vi "Field vs  IV_old_20180522.vi"() -> ()   [LabVIEW 2017]
uses:
  <vilib>/LabVIEW Targets/FPGA/cRIO/shared/nicrio_ModuleControls/nicrio_cRIO-9775_RecordDataRates4ChansRing.ctl
  <vilib>/Utility/file.llb/Write Delimited Spreadsheet (DBL).vi
  global.vi
  <resource>/objmgr/ni.dex.rc
panel:
  out "Array":dbl[](array[numeric])
  in  "Tab Control":enum32{"Field", "cRIO"}(tab)
  in  "Ramp type":string(combo)="Around origin"
  in  "Ramp up first T":bool=TRUE
  in  "Field Origin V":dbl format="%#_13g"
  in  "Field step V":dbl=0.005 format="%#_13g"
  in  "Field Radius V":dbl=1.0 format="%#_13g"
  in  "Init Ramp Time s":dbl=10.0
  in  "FIeld Scale factor":dbl=10.0
  in  "Step Ramp Time s":dbl=1.0
  in  "KEITHLEY 2400 GPIB Address":string="22"
  in  "cRIO IP":string="//172.22.11.2"
  in  "Data buffer size":i32=1000
  in  "Record Data Rate":T1=200 items=["20.000 MS/s (NI 9775)"=1, "10.00 MS/s (NI 9775)"=2, "6.667 MS/s (NI 9775)"=3, "5.000 MS/s (NI 9775)"=4, "2.500 MS/s (NI 9775)"=8, "1.667 MS/s (NI 9775)"=12, "1.250 MS/s (NI 9775)"=16, "1.000 MS/s (NI 9775)"=20, "833.333 KS/s (NI 9775)"=24, "714.286 KS/s (NI 9775)"=28, "625.000 KS/s (NI 9775)"=32, "555.556 KS/s (NI 9775)"=36, "500.000 KS/s (NI 9775)"=40, "454.545 KS/s (NI 9775)"=44, "416.667 KS/s (NI 9775)"=48, "384.615 KS/s (NI 9775)"=52, "357.143 KS/s (NI 9775)"=56, "333.333 KS/s (NI 9775)"=60, "312.500 KS/s (NI 9775)"=64, "294.118 KS/s (NI 9775)"=68, "277.778 KS/s (NI 9775)"=72, "263.158 KS/s (NI 9775)"=76, "250.000 KS/s (NI 9775)"=80, "238.095 KS/s (NI 9775)"=84, "227.273 KS/s (NI 9775)"=88, "217.391 KS/s (NI 9775)"=92, "208.333 KS/s (NI 9775)"=96, "200.000 KS/s (NI 9775)"=100, "192.308 KS/s (NI 9775)"=104, "185.185 KS/s (NI 9775)"=108, "178.571 KS/s (NI 9775)"=112, "172.414 KS/s (NI 9775)"=116, "166.667 KS/s (NI 9775)"=120, "161.290 KS/s (NI 9775)"=124, "156.250 KS/s (NI 9775)"=128, "151.515 KS/s (NI 9775)"=132, "147.059 KS/s (NI 9775)"=136, "142.857 KS/s (NI 9775)"=140, "138.889 KS/s (NI 9775)"=144, "135.135 KS/s (NI 9775)"=148, "131.579 KS/s (NI 9775)"=152, "128.205 KS/s (NI 9775)"=156, "125.000 KS/s (NI 9775)"=160, "121.951 KS/s (NI 9775)"=164, "119.048 KS/s (NI 9775)"=168, "116.279 KS/s (NI 9775)"=172, "113.636 KS/s (NI 9775)"=176, "111.111 KS/s (NI 9775)"=180, "108.696 KS/s (NI 9775)"=184, "106.383 KS/s (NI 9775)"=188, "104.167 KS/s (NI 9775)"=192, "102.041 KS/s (NI 9775)"=196, "100.000 KS/s (NI 9775)"=200, "50.000 KS/s (NI 9775)"=400, "33.333 KS/s (NI 9775)"=600, "25.000 KS/s (NI 9775)"=800, "20.000 KS/s (NI 9775)"=1000, "16.667 KS/s (NI 9775)"=1200, "14.286 KS/s (NI 9775)"=1400, "12.500 KS/s (NI 9775)"=1600, "11.111 KS/s (NI 9775)"=1800, "10.000 KS/s (NI 9775)"=2000, "9.091 KS/s (NI 9775)"=2200, "8.333 KS/s (NI 9775)"=2400, "7.692 KS/s (NI 9775)"=2600, "7.143 KS/s (NI 9775)"=2800, "6.667 KS/s (NI 9775)"=3000, "6.250 KS/s (NI 9775)"=3200, "5.882 KS/s (NI 9775)"=3400, "5.556 KS/s (NI 9775)"=3600, "5.000 KS/s (NI 9775)"=4000, "4.762 KS/s (NI 9775)"=4200, "4.545 KS/s (NI 9775)"=4400, "4.348 KS/s (NI 9775)"=4600, "4.167 KS/s (NI 9775)"=4800, "4.000 KS/s (NI 9775)"=5000, "3.846 KS/s (NI 9775)"=5200, "3.571 KS/s (NI 9775)"=5600, "3.333 KS/s (NI 9775)"=6000, "3.125 KS/s (NI 9775)"=6400, "2.941 KS/s (NI 9775)"=6800, "2.778 KS/s (NI 9775)"=7200, "2.632 KS/s (NI 9775)"=7600, "2.500 KS/s (NI 9775)"=8000, "2.381 KS/s (NI 9775)"=8400, "2.273 KS/s (NI 9775)"=8800, "2.174 KS/s (NI 9775)"=9200, "2.083 KS/s (NI 9775)"=9600, "2.000 KS/s (NI 9775)"=10000, "1.923 KS/s (NI 9775)"=10400, "1.852 KS/s (NI 9775)"=10800, "1.786 KS/s (NI 9775)"=11200, "1.724 KS/s (NI 9775)"=11600, "1.667 KS/s (NI 9775)"=12000, "1.613 KS/s (NI 9775)"=12400, "1.563 KS/s (NI 9775)"=12800, "1.515 KS/s (NI 9775)"=13200, "1.471 KS/s (NI 9775)"=13600, "1.429 KS/s (NI 9775)"=14000, "1.389 KS/s (NI 9775)"=14400, "1.351 KS/s (NI 9775)"=14800, "1.316 KS/s (NI 9775)"=15200, "1.282 KS/s (NI 9775)"=15600, "1.250 KS/s (NI 9775)"=16000, "1.220 KS/s (NI 9775)"=16400, "1.190 KS/s (NI 9775)"=16800, "1.163 KS/s (NI 9775)"=17200, "1.136 KS/s (NI 9775)"=17600, "1.111 KS/s (NI 9775)"=18000, "1.087 KS/s (NI 9775)"=18400, "1.064 KS/s (NI 9775)"=18800, "1.042 KS/s (NI 9775)"=19200, "1.020 KS/s (NI 9775)"=19600, "1.000 KS/s (NI 9775)"=20000, "0.980 KS/s (NI 9775)"=20400, "0.962 KS/s (NI 9775)"=20800, "0.943 KS/s (NI 9775)"=21200, "0.926 KS/s (NI 9775)"=21600, "0.909 KS/s (NI 9775)"=22000, "0.893 KS/s (NI 9775)"=22400, "0.877 KS/s (NI 9775)"=22800, "0.862 KS/s (NI 9775)"=23200, "0.847 KS/s (NI 9775)"=23600, "0.833 KS/s (NI 9775)"=24000, "0.820 KS/s (NI 9775)"=24400, "0.806 KS/s (NI 9775)"=24800, "0.794 KS/s (NI 9775)"=25200, "0.781 KS/s (NI 9775)"=25600, "0.694 KS/s (NI 9775)"=28800, "0.625 KS/s (NI 9775)"=32000, "0.568 KS/s (NI 9775)"=35200, "0.521 KS/s (NI 9775)"=38400, "0.446 KS/s (NI 9775)"=44800, "0.391 KS/s (NI 9775)"=51200, "0.347 KS/s (NI 9775)"=57600, "0.313 KS/s (NI 9775)"=64000]
  in  "Gate wait time us":u32=150
  in  "Record Samples":u32=5000
  in  "Current Scale factor":dbl=5.0
  in  "Average num":i32=10
  in  "Voltage Scale factor":dbl=0.0001
  in  "Stop loop":bool
  out "Current Field mT":dbl=-0.050000000000000044
  out "Current Field V":dbl=-0.0050000000000000044
  in  "Name":string="book381"
  in  "Contour plot folder":path=path "C:/Users/gyue/Box Sync/Guang Yue/data/Contour plot"
  out "IV parameters":T2={"Records Num"=1, "AI Trigger Configuration"={"Trigger Slope"=enum."Positive", "Trigger Level"=0.10009765625, "Hystesis Value"=0.094970703125, "AI Channel"=0}, "Record PreTrigger Samples"=1, "Record Samples"=5000, "Ic Cut off or curve"=FALSE, "Gate wait time us"=150, "Record Data Rate"=200} {"Record Data Rate" items=["20.000 MS/s (NI 9775)"=1, "10.00 MS/s (NI 9775)"=2, "6.667 MS/s (NI 9775)"=3, "5.000 MS/s (NI 9775)"=4, "2.500 MS/s (NI 9775)"=8, "1.667 MS/s (NI 9775)"=12, "1.250 MS/s (NI 9775)"=16, "1.000 MS/s (NI 9775)"=20, "833.333 KS/s (NI 9775)"=24, "714.286 KS/s (NI 9775)"=28, "625.000 KS/s (NI 9775)"=32, "555.556 KS/s (NI 9775)"=36, "500.000 KS/s (NI 9775)"=40, "454.545 KS/s (NI 9775)"=44, "416.667 KS/s (NI 9775)"=48, "384.615 KS/s (NI 9775)"=52, "357.143 KS/s (NI 9775)"=56, "333.333 KS/s (NI 9775)"=60, "312.500 KS/s (NI 9775)"=64, "294.118 KS/s (NI 9775)"=68, "277.778 KS/s (NI 9775)"=72, "263.158 KS/s (NI 9775)"=76, "250.000 KS/s (NI 9775)"=80, "238.095 KS/s (NI 9775)"=84, "227.273 KS/s (NI 9775)"=88, "217.391 KS/s (NI 9775)"=92, "208.333 KS/s (NI 9775)"=96, "200.000 KS/s (NI 9775)"=100, "192.308 KS/s (NI 9775)"=104, "185.185 KS/s (NI 9775)"=108, "178.571 KS/s (NI 9775)"=112, "172.414 KS/s (NI 9775)"=116, "166.667 KS/s (NI 9775)"=120, "161.290 KS/s (NI 9775)"=124, "156.250 KS/s (NI 9775)"=128, "151.515 KS/s (NI 9775)"=132, "147.059 KS/s (NI 9775)"=136, "142.857 KS/s (NI 9775)"=140, "138.889 KS/s (NI 9775)"=144, "135.135 KS/s (NI 9775)"=148, "131.579 KS/s (NI 9775)"=152, "128.205 KS/s (NI 9775)"=156, "125.000 KS/s (NI 9775)"=160, "121.951 KS/s (NI 9775)"=164, "119.048 KS/s (NI 9775)"=168, "116.279 KS/s (NI 9775)"=172, "113.636 KS/s (NI 9775)"=176, "111.111 KS/s (NI 9775)"=180, "108.696 KS/s (NI 9775)"=184, "106.383 KS/s (NI 9775)"=188, "104.167 KS/s (NI 9775)"=192, "102.041 KS/s (NI 9775)"=196, "100.000 KS/s (NI 9775)"=200, "50.000 KS/s (NI 9775)"=400, "33.333 KS/s (NI 9775)"=600, "25.000 KS/s (NI 9775)"=800, "20.000 KS/s (NI 9775)"=1000, "16.667 KS/s (NI 9775)"=1200, "14.286 KS/s (NI 9775)"=1400, "12.500 KS/s (NI 9775)"=1600, "11.111 KS/s (NI 9775)"=1800, "10.000 KS/s (NI 9775)"=2000, "9.091 KS/s (NI 9775)"=2200, "8.333 KS/s (NI 9775)"=2400, "7.692 KS/s (NI 9775)"=2600, "7.143 KS/s (NI 9775)"=2800, "6.667 KS/s (NI 9775)"=3000, "6.250 KS/s (NI 9775)"=3200, "5.882 KS/s (NI 9775)"=3400, "5.556 KS/s (NI 9775)"=3600, "5.000 KS/s (NI 9775)"=4000, "4.762 KS/s (NI 9775)"=4200, "4.545 KS/s (NI 9775)"=4400, "4.348 KS/s (NI 9775)"=4600, "4.167 KS/s (NI 9775)"=4800, "4.000 KS/s (NI 9775)"=5000, "3.846 KS/s (NI 9775)"=5200, "3.571 KS/s (NI 9775)"=5600, "3.333 KS/s (NI 9775)"=6000, "3.125 KS/s (NI 9775)"=6400, "2.941 KS/s (NI 9775)"=6800, "2.778 KS/s (NI 9775)"=7200, "2.632 KS/s (NI 9775)"=7600, "2.500 KS/s (NI 9775)"=8000, "2.381 KS/s (NI 9775)"=8400, "2.273 KS/s (NI 9775)"=8800, "2.174 KS/s (NI 9775)"=9200, "2.083 KS/s (NI 9775)"=9600, "2.000 KS/s (NI 9775)"=10000, "1.923 KS/s (NI 9775)"=10400, "1.852 KS/s (NI 9775)"=10800, "1.786 KS/s (NI 9775)"=11200, "1.724 KS/s (NI 9775)"=11600, "1.667 KS/s (NI 9775)"=12000, "1.613 KS/s (NI 9775)"=12400, "1.563 KS/s (NI 9775)"=12800, "1.515 KS/s (NI 9775)"=13200, "1.471 KS/s (NI 9775)"=13600, "1.429 KS/s (NI 9775)"=14000, "1.389 KS/s (NI 9775)"=14400, "1.351 KS/s (NI 9775)"=14800, "1.316 KS/s (NI 9775)"=15200, "1.282 KS/s (NI 9775)"=15600, "1.250 KS/s (NI 9775)"=16000, "1.220 KS/s (NI 9775)"=16400, "1.190 KS/s (NI 9775)"=16800, "1.163 KS/s (NI 9775)"=17200, "1.136 KS/s (NI 9775)"=17600, "1.111 KS/s (NI 9775)"=18000, "1.087 KS/s (NI 9775)"=18400, "1.064 KS/s (NI 9775)"=18800, "1.042 KS/s (NI 9775)"=19200, "1.020 KS/s (NI 9775)"=19600, "1.000 KS/s (NI 9775)"=20000, "0.980 KS/s (NI 9775)"=20400, "0.962 KS/s (NI 9775)"=20800, "0.943 KS/s (NI 9775)"=21200, "0.926 KS/s (NI 9775)"=21600, "0.909 KS/s (NI 9775)"=22000, "0.893 KS/s (NI 9775)"=22400, "0.877 KS/s (NI 9775)"=22800, "0.862 KS/s (NI 9775)"=23200, "0.847 KS/s (NI 9775)"=23600, "0.833 KS/s (NI 9775)"=24000, "0.820 KS/s (NI 9775)"=24400, "0.806 KS/s (NI 9775)"=24800, "0.794 KS/s (NI 9775)"=25200, "0.781 KS/s (NI 9775)"=25600, "0.694 KS/s (NI 9775)"=28800, "0.625 KS/s (NI 9775)"=32000, "0.568 KS/s (NI 9775)"=35200, "0.521 KS/s (NI 9775)"=38400, "0.446 KS/s (NI 9775)"=44800, "0.391 KS/s (NI 9775)"=51200, "0.347 KS/s (NI 9775)"=57600, "0.313 KS/s (NI 9775)"=64000]}
  out "IV curve":cluster{"Y":dbl[], "Y":dbl[]}[](graph)
  in  "stop":bool
  out "error out":errorcluster={"status"=FALSE, "code"=180121605, "source"="Shared Variable in Field vs  IV.vi<APPEND>\nThis error or warning occurred while writing the following Shared Variable:\n\\\\NI-cRIO-9063-01bc8cc6\\network varibles\\RT Stop\n\\\\172.22.11.2\\network varibles\\RT Stop"}
  # "Voltage x factor=mT"
  # "Voltage x factor=uA"
  # "Voltage x factor=uA"
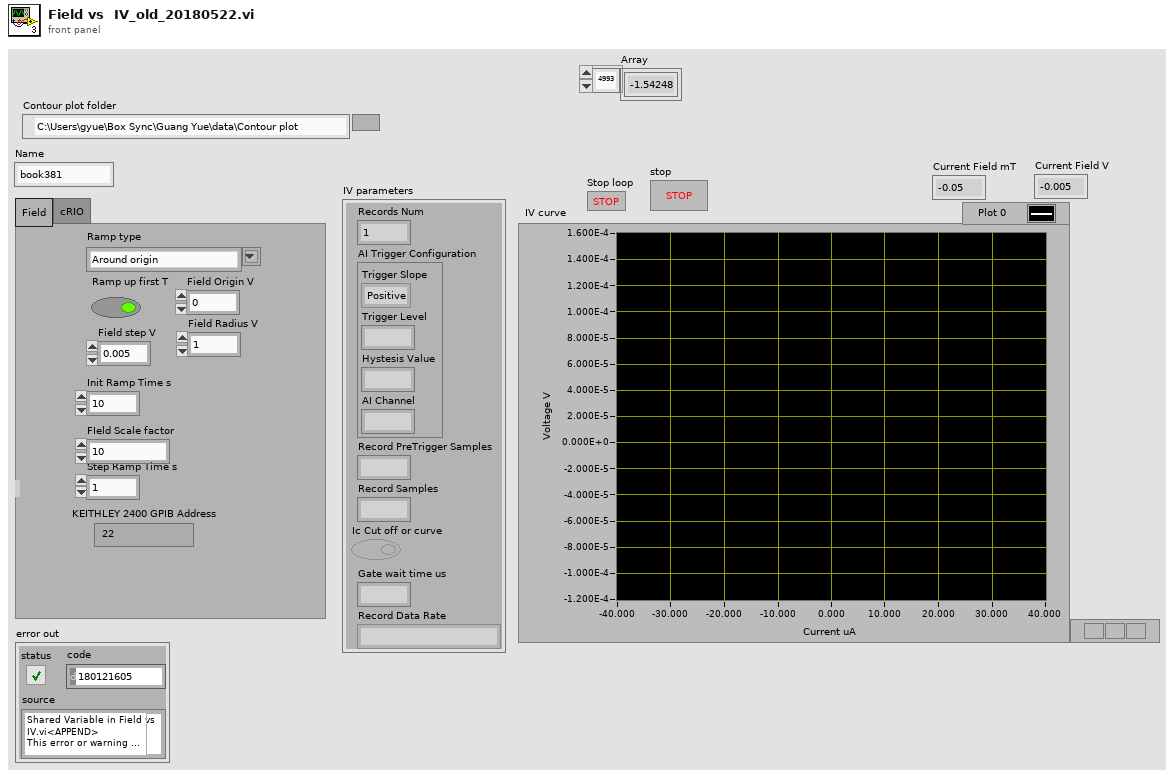
[diagram p1: front panel]
types:
  T1 = typedef "nicrio_cRIO-9775_RecordDataRates4ChansRing.ctl" = u16
  T2 = cluster{"Records Num":i32, "AI Trigger Configuration":cluster{"Trigger Slope":enum8{"Positive", "Negative"}, "Trigger Level":fxp<+/-,17,5>, "Hystesis Value":fxp<+,16,4>, "AI Channel":u8}, "Record PreTrigger Samples":u32, "Record Samples":u32, "Ic Cut off or curve":bool, "Gate wait time us":u32, "Record Data Rate":T1}
  T3 = cluster{"Trigger Slope":enum8{"Positive", "Negative"}, "Trigger Level":fxp<+/-,17,5>, "Hystesis Value":fxp<+,16,4>, "AI Channel":u8}
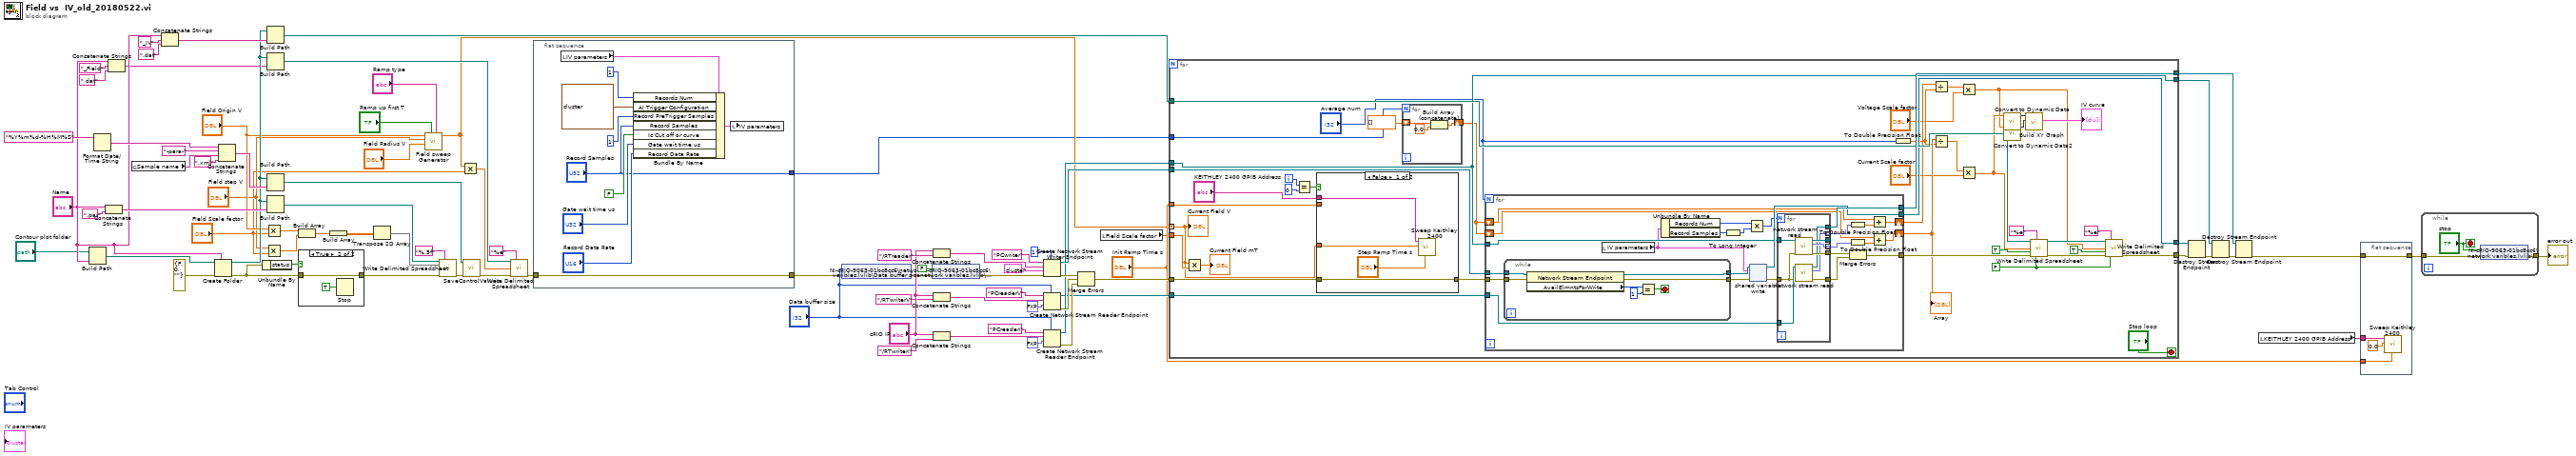
[diagram p0: block diagram]
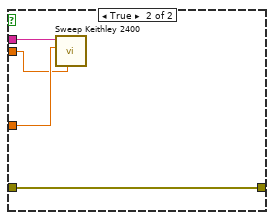
[diagram p3: hidden frame]
diagram:
  n1 = Build Path(base path="Contour plot folder", name or relative path="Name") -> (appended path=w37:path)
  n2 = Format Date/Time String(time format string (%c)="%Y%m%d-%H%M%S") -> (date/time string=w32:string)  [unwired: 2 in]
  n3 = Concatenate Strings("Name", ".par" ("string")) -> (w44:string)
  n4 = Concatenate Strings("Name", "_Field" ("string"), ".dat" ("string")) -> (w21:string)
  n5 = global read "global.vi" "Sample name"() -> (w31:string)
  n6 = Concatenate Strings("Name", "_IV" ("string"), ".dat" ("string")) -> (w38:string)
  n7 = Create Folder(prompt (Create Folder)="Name", path (use dialog)=w37, error in=errorcluster {"status"=FALSE, "code"=0, "source"=""}) -> (created path=w22:path, error out=w34:errorcluster)  [unwired: 1 out]
  n8 = Concatenate Strings(w32, "-para-" ("string"), w31, ".xml" ("string")) -> (w48:string)
  n9 = Unbundle By Name(w34) -> ("status"=w35:bool)
  n10 = Multiply(x="Field Origin V", y="FIeld Scale factor") -> (x*y=w30:dbl)
  n11 = Multiply(x="Field step V", y="FIeld Scale factor") -> (x*y=w29:dbl)
  n12 = Build Path(base path=w22, name or relative path=w38) -> (appended path=w20:path)
  n13 = Build Path(base path=w22, name or relative path=w21) -> (appended path=w9:path)
  n14 = Build Path(base path=w22, name or relative path=w48) -> (appended path=w46:path)
  n15 = Build Path(base path=w22, name or relative path=w44) -> (appended path=w43:path)
  n16 = Build Array(w30, w29) -> (w41:dbl[])
  n17 = case shown="True" w35 {
    tunnel: [w84 w86] -> w33
    tunnel: w34 -> [w84 w86]
    frame False {
    }
    frame True {
      n18 = Stop(stop? (T)=TRUE) -> ()
    }
  }
  n19 = Build Array(w41) -> (w40:dbl[][])
  n20 = Transpose 2D Array(2D array=w40) -> (transposed array=w39:dbl[][])
  n21 = call "Field sweep Generator.vi"("Ramp type"="Ramp type", "Ramp up first T"="Ramp up first T", "Field Radius V"="Field Radius V", "Field step V"="Field step V", "Field Origin V"="Field Origin V") -> ("output array"=w4:dbl[])  [unwired: 6 in]
  n22 = call-poly <vilib>:"Write Delimited Spreadsheet.vi"("file path (dialog if empty)"=w43, "format (%.3f)"="%.5f", "2D data"=w39, "error in (no error)"=w33) -> ("error out"=w36:errorcluster)  [unwired: 10 in, 1 out]
  n23 = Multiply(x=w4, y="FIeld Scale factor") -> (x*y=w7:dbl[])
  n24 = call "SaveControlValues.vi"("XML File Path"=w46, "error in (no error)"=w36) -> ("error out"=w6:errorcluster)  [unwired: 8 in]
  n25 = call-poly <vilib>:"Write Delimited Spreadsheet.vi"("file path (dialog if empty)"=w9, "format (%.3f)"="%e", "1D data"=w7, "error in (no error)"=w6) -> ("error out"=w3:errorcluster)  [unwired: 10 in, 1 out]
  n26 = flat-sequence {
    tunnel: w3 -> [w96]
    tunnel: [w96] -> w2
    tunnel: ["Record Samples"] -> w1
    frame #0 {
      n27 = local read "IV parameters"() -> (w95:T2)
      n28 = Bundle By Name(cluster=w95, "Records Num"=1, "AI Trigger Configuration"=T3 {"Trigger Slope"=enum."Positive", "Trigger Level"=0.10009765625, "Hystesis Value"=0.094970703125, "AI Channel"=0}, "Record PreTrigger Samples"=u32 1, "Record Samples"="Record Samples", "Ic Cut off or curve"=FALSE, "Gate wait time us"="Gate wait time us", "Record Data Rate"="Record Data Rate") -> (w89:T2)
      n29 = local write "IV parameters"(w89) -> ()
    }
  }
  n30 = shared-variable "NI-cRIO-9063-01bc8cc6\\network varibles.lvlib\\Data buffer size"("Data buffer size", error in=w2) -> (error out=w61:errorcluster)
  n31 = shared-variable "NI-cRIO-9063-01bc8cc6\\network varibles.lvlib\\RT Stop"(FALSE ("RT Stop"), error in=w61) -> (error out=w69:errorcluster)
  n32 = Concatenate Strings("cRIO IP", "/RTreader" ("string")) -> (w79:string)
  n33 = Concatenate Strings("cRIO IP", "/RTwriterV" ("string")) -> (w71:string)
  n34 = Concatenate Strings("cRIO IP", "/RTwriterI" ("string")) -> (w63:string)
  n35 = Create Network Stream Writer Endpoint(7:1 ("writer buffer size"), 8:w69, 9:T2 {"Records Num"=0, "AI Trigger Configuration"={"Trigger Slope"=enum."Positive", "Trigger Level"=0.0, "Hystesis Value"=0.0, "AI Channel"=0}, "Record PreTrigger Samples"=0, "Record Samples"=0, "Ic Cut off or curve"=FALSE, "Gate wait time us"=0, "Record Data Rate"=1} ("Parameters 4"), 10:w79, 11:"PCwriter" ("writer name")) -> (0:w77:errorcluster, 3:w76:refnum<k21>)  [unwired: 2 in]
  n36 = Create Network Stream Reader Endpoint(7:"Data buffer size", 9:fxp<+/-,17,5> 0.0, 10:w71, 11:"PCreaderV" ("reader name")) -> (0:w68:errorcluster, 3:w55:refnum<k21>)  [unwired: 3 in]
  n37 = Create Network Stream Reader Endpoint(7:"Data buffer size", 9:fxp<+/-,17,5> 0.0, 10:w63, 11:"PCreaderI" ("reader name")) -> (0:w60:errorcluster, 3:w58:refnum<k21>)  [unwired: 3 in]
  n38 = Merge Errors(w77, w68, w60) -> (w75:errorcluster)
  n39 = local read "FIeld Scale factor"() -> (w5:dbl)
  n40 = for {
    tunnel: w76 -> [w138]
    tunnel: [w123] -> w56
    tunnel: w75 -> [w128]
    tunnel: [w121] -> w53
    tunnel: w58 -> [w122]
    tunnel: [w122] -> w57
    tunnel: w55 -> [w137]
    tunnel: [w136] -> w54
    tunnel: w5 -> [w132]
    tunnel: "Init Ramp Time s" -> [w129]
    tunnel: w20 -> [w126]
    tunnel: w4 -> [w124] mode=indexing
    tunnel: w1 -> [w99]
    i -> [w133]
    stop <- "Stop loop" stop-if-true
    w108 = FALSE ("transpose? (no:F)")
    n41 = Multiply(x=w124, y=w132) -> (x*y=→"Current Field mT":dbl)
    n42 = Equal?(x=w133, y=0) -> (x = y?=w131:bool)
    n43 = case shown="False" w131 {
      tunnel: w128 -> [w186 w187]
      tunnel: [w186 w187] -> w127
      tunnel: w124 -> [w183 w190]
      tunnel: "KEITHLEY 2400 GPIB Address" -> [w184 w189]
      tunnel: w129 -> [_ w188]
      frame False {
        n44 = call "Sweep Keithley 2400.vi"("Ramp Time (s)"="Step Ramp Time s", "final gate voltage (V)"=w183, "KEITHLEY 2400 GPIB Address"=w184) -> ()  [unwired: 7 in, 2 out]
      }
      frame True {
        n45 = call "Sweep Keithley 2400.vi"("Ramp Time (s)"=w188, "final gate voltage (V)"=w190, "KEITHLEY 2400 GPIB Address"=w189) -> ()  [unwired: 7 in, 2 out]
      }
    }
    n46 = for {
      N: w99 -> [_]
      shift-right: [w140] -> w100
      shift-left: dbl[] [] -> [w141]
      n47 = Build Array (concatenate)(w141, 0.0 ("new element/subarray")) -> (w140:dbl[])
    }
    n48 = for {
      N: "Average num" -> [_]
      tunnel: w122 -> [w161]
      tunnel: w138 -> [w166]
      tunnel: [w162] -> w123
      tunnel: w137 -> [w165]
      tunnel: [w164] -> w136
      tunnel: w127 -> [w163]
      tunnel: [w150] -> w115
      shift-right: [w145] -> w109
      shift-left: w100 -> [w147]
      shift-right: [w143] -> w110
      shift-left: w100 -> [w142]
      n49 = while {
        tunnel: w166 -> [w182]
        tunnel: w163 -> [w181]
        tunnel: [w177] -> w160
        tunnel: [w176] -> w159
        stop <- w178 stop-if-true
        n50 = property class="Network Stream Endpoint"(reference=w182, error in=w181) -> (reference out=w177:refnum<k21>, error out=w176:errorcluster, "AvailElmntsForWrite"=w180:i32)
        n51 = Equal?(x=w180, y=1) -> (x = y?=w178:bool)
      }
      n52 = local read "IV parameters"() -> (w157:T2)
      n53 = Unbundle By Name(w157) -> ("Records Num"=w156:i32, "Record Samples"=w155:u32)
      n54 = To Long Integer(number=w155) -> (32bit integer=w154:i32)
      n55 = Multiply(x=w156, y=w154) -> (x*y=w153:i32)
      n56 = shared-variable-write(w160, w159, w157) -> (w162:refnum<k21>, w158:errorcluster)  [unwired: 1 in, 1 out]
      n57 = for {
        N: w153 -> [_]
        tunnel: w161 -> [w175]
        tunnel: w158 -> [w168]
        tunnel: [w174] -> w149 mode=indexing
        tunnel: [w173] -> _
        tunnel: [w172] -> w152
        tunnel: w165 -> [w171]
        tunnel: [w170] -> w164
        tunnel: [w169] -> w148 mode=indexing
        tunnel: [w167] -> w151
        n58 = call "network stream read.vi"("error in (no error)"=w168, "endpoint in"=w175) -> ("error out"=w172:errorcluster, "Data"=w174:fxp<+/-,17,5>, "endpoint out"=w173:refnum<k21>)  [unwired: 7 in]
        n59 = call "network stream read.vi"("error in (no error)"=w168, "endpoint in"=w171) -> ("error out"=w167:errorcluster, "Data"=w169:fxp<+/-,17,5>, "endpoint out"=w170:refnum<k21>)  [unwired: 7 in]
      }
      n60 = To Double Precision Float(number=w148) -> (double precision float=w146:dbl[])
      n61 = To Double Precision Float(number=w149) -> (double precision float=w144:dbl[])
      n62 = Merge Errors(w152, w151) -> (w150:errorcluster)
      n63 = Add(x=w147, y=w146) -> (x+y=w145:dbl[])
      n64 = Add(x=w142, y=w144) -> (x+y=w143:dbl[])
    }
    "Array" <- w110
    n65 = To Double Precision Float(number="Average num") -> (double precision float=w107:dbl)
    n66 = Divide(x=w109, y=w107) -> (x/y=w104:dbl[])
    n67 = Divide(x=w110, y=w107) -> (x/y=w105:dbl[])
    n68 = Multiply(x=w104, y="Voltage Scale factor") -> (x*y=w97:dbl[])
    n69 = Multiply(x=w105, y="Current Scale factor") -> (x*y=w98:dbl[])
    n70 = call "Convert to Dynamic Data"("Array"=w98) -> ("Dynamic Data Type"=w119:dynamicdata)  [unwired: 3 in]
    n71 = call "Convert to Dynamic Data2"("Array"=w97) -> ("Dynamic Data Type"=w118:dynamicdata)  [unwired: 3 in]
    n72 = call "Build XY Graph"("Y Input"=w118, "X Input"=w119) -> ("XY Graph"=→"IV curve":cluster{"X":dbl[], "Y":dbl[]}[])  [unwired: 8 in, 1 out]
    n73 = call-poly <vilib>:"Write Delimited Spreadsheet.vi"("file path (dialog if empty)"=w126, "format (%.3f)"="%e", "1D data"=w98, "append to file? (new file:F)"=TRUE, "error in (no error)"=w115, "transpose? (no:F)"=w108) -> ("new file path (Not A Path if cancelled)"=w111:path, "error out"=w112:errorcluster)  [unwired: 8 in]
    n74 = call-poly <vilib>:"Write Delimited Spreadsheet.vi"("file path (dialog if empty)"=w111, "format (%.3f)"="%e", "1D data"=w97, "append to file? (new file:F)"=TRUE, "error in (no error)"=w112, "transpose? (no:F)"=w108) -> ("error out"=w121:errorcluster)  [unwired: 8 in, 1 out]
    "Current Field V" <- w124
  }
  n75 = Destroy Stream Endpoint(8:w53, 11:w56) -> (0:w67:errorcluster)
  n76 = Destroy Stream Endpoint(8:w67, 11:w57) -> (0:w59:errorcluster)
  n77 = Destroy Stream Endpoint(8:w59, 11:w54) -> (0:w16:errorcluster)
  n78 = local read "KEITHLEY 2400 GPIB Address"() -> (w17:string)
  n79 = flat-sequence {
    tunnel: w16 -> [w194]
    tunnel: [w194] -> w19
    tunnel: "Init Ramp Time s" -> [w193]
    tunnel: w17 -> [w191]
    frame #0 {
      n80 = call "Sweep Keithley 2400.vi"("Ramp Time (s)"=w193, "final gate voltage (V)"=0.0, "KEITHLEY 2400 GPIB Address"=w191) -> ()  [unwired: 7 in, 2 out]
    }
  }
  n81 = while {
    tunnel: w19 -> [w196]
    tunnel: [w195] -> w66
    stop <- "stop" stop-if-true
    n82 = shared-variable "NI-cRIO-9063-01bc8cc6\\network varibles.lvlib\\RT Stop"("stop", error in=w196) -> (error out=w195:errorcluster)
  }
  "error out" <- w66
